vi "CalcularArea.vi"(8 "error in":errorcluster, 11 "object in":refnum<class "Rectangulo.lvclass">) -> (0 "error out":errorcluster, 2 "Area":dbl, 3 "object out":refnum<class "Rectangulo.lvclass">)   [LabVIEW 2024, in "Rectangulo.lvclass"]
uses:
  Rectangulo.lvclass
  Rectangulo.lvclass/Rectangulo.ctl
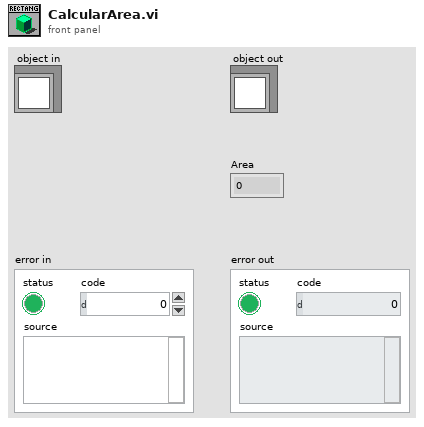
[diagram p1: front panel]
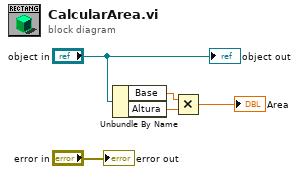
[diagram p0: block diagram]
diagram:
  n1 = Unbundle By Name("object in") -> ("Base"=w3:dbl, "Altura"=w2:dbl)
  n2 = Multiply(x=w3, y=w2) -> (x*y=→"Area":dbl)
  "error out" <- "error in"
  "object out" <- "object in"
